vi "SPECAN_AMPM_ACP_TXP.vi"() -> ()   [LabVIEW 2016]
doc: "This example illustrates how to use the RFmx SpecAn and LTE personalities together with the RFSG drivers to perform ACP and EVM measurements with or without digital predistortion (DPD) of the waveform input to the DUT. \n\nDPD is a technique to optimize the operating point of power amplifiers and other non-linear RFIC devices. Power amplifiers are much more efficient if they operate near compression. However, compressing signal amplitudes can significantly deteriorate the amplified signal's quality both, in-band (e.g., EVM increases due to non-linear distortion of the signal's I/Q constellation) and out-of-band (e.g., ACP or SEM test fails due to spectral regrowth). With DPD, the original waveform is first pre-distorted in a way that matches the non-linear effects of the RFIC device before being fed through the device. The resulting output is a much cleaner amplified and/or filtered version of the original waveform. \n\nDifferent DPD models can be used to trade off performance with computational ease, with the Lookup-Table (LUT) model the simplest and the Generalized Memory Polynomial Model (GMP) the most complex. With a LUT, the DPD algorithm achieves gain and phase linearization on average. If you want to correct for memory effects - i.e., an output sample not only depends on the current input but also previous input samples; you will notice that a specific input power value translates into a range of gain and phase values - you would use one of the memory polynomial models. For these models, several parameters such as polynomial order and memory depth are available to fine-tune the model to the DUT behavior."
uses:
  <instrlib>/niRFSG/niRFSG.llb/niRFSG Exported Signal Destinations.ctl
  Source/SG/Typedefs/Instrument Configuration.ctl
  <instrlib>/niRFSG/niRFSG.llb/niRFSG Ref Clock Sources.ctl
  Source/SA/RFmxSpecAn/Typedefs/SpecAn AMPM Configuration.ctl
  Source/SG/Typedefs/Waveform.ctl
  Source/SA/RFmxSpecAn/Typedefs/SpecAn AMPM Results.ctl
  Source/SA/RFmxSpecAn/Typedefs/SpecAn Common Configuration.ctl
  Source/SA/RFmxSpecAn/Typedefs/SpecAn ACP Configuration.ctl
  Source/SA/RFmxSpecAn/Typedefs/SpecAn ACP Carrier Channel Configuration.ctl
  Source/SA/RFmxSpecAn/Typedefs/SpecAn ACP Offset Channel Configuration.ctl
  Source/SA/RFmxSpecAn/Typedefs/SpecAn ACP Offset Results.ctl
  Source/SA/RFmxSpecAn/Typedefs/SpecAn ACP Component Carrier Results.ctl
  Source/SA/RFmxSpecAn/Typedefs/SpecAn TxP Configuration.ctl
  Source/SA/RFmxSpecAn/Typedefs/SpecAn TxP Results.ctl
  <vilib>/RFmx/SpecAn/mx/RFmxSpecAn.llb/RFmxSpecAn Select Measurement (Single).vi
  <vilib>/RFmx/SpecAn/mx/RFmxSpecAn.llb/RFmxSpecAn AMPM Fetch AM to AM Trace.vi
  <vilib>/RFmx/SpecAn/mx/RFmxSpecAn.llb/RFmxSpecAn AMPM Fetch AM to PM Trace.vi
  <vilib>/RFmx/SpecAn/mx/RFmxSpecAn.llb/RFmxSpecAn ACP Fetch Spectrum.vi
  <vilib>/RFmx/SpecAn/mx/RFmxSpecAn.llb/RFmxSpecAn TXP Fetch Power Trace.vi
  Source/SG/SG.lvlib
  Source/SA/RFmxSpecAn/RFmxSpecAn.lvlib
panel:
  in  "Display Tab Control":enum32{"AMPM Results", "ACP Results", "TxP"}(tab)
  out "AM to AM Plot":T1(graph)
  out "AM to PM Plot":T2(graph)
  out "AMPM Measurement Results":T3 {"AM to PM Residual (deg)" format="%.2f"; "AM to AM Residual (dB)" format="%.2f"; "Mean RMS EVM (%)" format="%.2f"; "1 dB Compression Point (dBm)" format="%.2f"; "Mean Linear Gain (dB)" format="%.2f"}
  out "Spectrum":cluster{"x0":dbl, "dx":dbl, "y":sgl[]}(graph) caption="DUT Output Spectrum"
  out "Offset Results":T4[](array[typedef])
  out "Component Carrier Results":T5[](array[typedef])
  out "Total Carrier Power (dBm or dBm/Hz)":dbl
  out "Power Trace":cluster{"x0":dbl, "dx":dbl, "y":sgl[]}(graph)
  out "TxP Results":T6 {"Minimum Power (dBm)" format="%.2f"; "Maximum Power (dBm)" format="%.2f"; "Peak to Average Ratio (dB)" format="%.2f"; "Average Mean Power (dBm)" format="%.2f"}
  in  "Measurement Settings Tab Control":T7(tab)
  in  "TxP Config":T8={"Measurement Interval (s)"=0.001, "RBW (Hz)"=20000000.0, "RBW Filter Type"=5, "RRC Alpha"=0.0, "Averaging Enabled"=0, "Averaging Count"=10, "Averaging Type"=0} {"Averaging Type" items=["RMS", "Log", "Scalar", "Max", "Min"]; "Averaging Enabled" items=["False", "True"]; "RRC Alpha" format="%.3g"; "RBW Filter Type" items=["None"=5, "Gaussian"=1, "Flat"=2, "RRC"=6]; "RBW (Hz)" format="%.3p"; "Measurement Interval (s)" format="%.2p"}
  in  "RFmx SpecAn AMPM Configuration":T9={"Measurement Interval (s)"=0.0001, "DUT Average Input Power (dBm)"=-20.0, "Signal Type"=0, "Reference Waveform"={"Waveform Name"="Wfm", "Waveform"={"x0"=0.0, "dx"=0.0, "y"=[]}, "Signal Bandwidth (Hz)"=0.0, "PAPR (dB)"=0.0, "Burst Length (s)"=0.0, "Sample Rate"=0.0, "Burst Start Locations"=[], "Burst Stop Locations"=[], "Idle Duration Present?"=FALSE, "Runtime Scaling"=0.0}} {"Reference Waveform"."Runtime Scaling" format="%#_6p"; "Reference Waveform"."Sample Rate" format="%#_6p"; "Reference Waveform"."Burst Length (s)" format="%#_6p"; "Reference Waveform"."PAPR (dB)" format="%.2f"; "Reference Waveform"."Signal Bandwidth (Hz)" format="%#_6p"; "Reference Waveform"."Waveform"."y" format="%.2f"; "Reference Waveform"."Waveform"."dx" format="%^.2e"; "Reference Waveform"."Waveform"."x0" format="%^.2e"; "Signal Type" items=["Modulated", "Tones"]; "DUT Average Input Power (dBm)" format="%.2f"; "Measurement Interval (s)" format="%.2p"}
  in  "ACP Configuration":T11={"Power Units"=0, "Averaging Enabled"=0, "Averaging Count"=10, "Averaging Type"=0, "FFT Window"=1, "FFT Padding"=-1.0, "RBW Auto"=1, "RBW (Hz)"=10000.0, "RBW Filter Type"=1, "Sweep Time Auto"=1, "Sweep Time Interval (s)"=0.001, " Carrier Channel Configuration"=[], "Offset Channel Configuration"=[]} {"Offset Channel Configuration"."RRC Alpha" format="%.3g"; "Offset Channel Configuration"."RRC Filter Enabled" items=["False", "True"]; "Offset Channel Configuration"."Relative Attenuation (dB)" format="%.2f"; "Offset Channel Configuration"."Power Reference Carrier" items=["Closest", "Highest", "Composite", "Specific"]; "Offset Channel Configuration"."Sideband" items=["Neg", "Pos", "Both"]; "Offset Channel Configuration"."Frequency (Hz)" format="%.3p"; "Offset Channel Configuration"."Enabled" items=["False", "True"]; "Offset Channel Configuration"."Integration Bandwidth (Hz)" format="%.3p"; "Carrier Channel Configuration"."RRC Alpha" format="%.3g"; "Carrier Channel Configuration"."RRC Filter Enabled" items=["False", "True"]; "Carrier Channel Configuration"."Mode" items=["Passive", "Active"]; "Carrier Channel Configuration"."Frequency (Hz)" format="%.3p"; "Carrier Channel Configuration"."Integration Bandwidth (Hz)" format="%.3p"; "Sweep Time Interval (s)" format="%.2p"; "Sweep Time Auto" items=["False", "True"]; "RBW Filter Type" items=["FFT Based", "Gaussian", "Flat", "Synch Tuned - 4", "Synch Tuned - 5"]; "RBW (Hz)" format="%.3p"; "RBW Auto" items=["False", "True"]; "FFT Padding" format="%.2f"; "FFT Window" items=["None", "Flat Top", "Hanning", "Hamming", "Gaussian", "Blackman", "Blackman-Harris", "Kaiser-Bessel"]; "Averaging Type" items=["RMS", "Log", "Scalar", "Max", "Min", "Vector"]; "Averaging Enabled" items=["False", "True"]; "Power Units" items=["dBm", "dBm/Hz"]}
  in  "Offset Channel Configuration":T13[](array[typedef])=[{"Integration Bandwidth (Hz)"=18000000.0, "Enabled"=1, "Frequency (Hz)"=20000000.0, "Sideband"=2, "Power Reference Carrier"=0, "Power Reference Specific Index"=0, "Relative Attenuation (dB)"=0.0, "RRC Filter Enabled"=0, "RRC Alpha"=0.22}, {"Integration Bandwidth (Hz)"=3840000.0, "Enabled"=1, "Frequency (Hz)"=12500000.0, "Sideband"=2, "Power Reference Carrier"=0, "Power Reference Specific Index"=0, "Relative Attenuation (dB)"=0.0, "RRC Filter Enabled"=0, "RRC Alpha"=0.22}, {"Integration Bandwidth (Hz)"=3840000.0, "Enabled"=1, "Frequency (Hz)"=17500000.0, "Sideband"=2, "Power Reference Carrier"=0, "Power Reference Specific Index"=0, "Relative Attenuation (dB)"=0.0, "RRC Filter Enabled"=0, "RRC Alpha"=0.22}] {"RRC Alpha" format="%.3g"; "RRC Filter Enabled" items=["False", "True"]; "Relative Attenuation (dB)" format="%.2f"; "Power Reference Carrier" items=["Closest", "Highest", "Composite", "Specific"]; "Sideband" items=["Neg", "Pos", "Both"]; "Frequency (Hz)" format="%.3p"; "Enabled" items=["False", "True"]; "Integration Bandwidth (Hz)" format="%.3p"}
  in  "Carrier Channel Configuration":T12[](array[typedef])=[{"Frequency (Hz)"=0.0, "Integration Bandwidth (Hz)"=18000000.0, "Mode"=1, "RRC Filter Enabled"=0, "RRC Alpha"=0.22}] {"RRC Alpha" format="%.3g"; "RRC Filter Enabled" items=["False", "True"]; "Mode" items=["Passive", "Active"]; "Frequency (Hz)" format="%.3p"; "Integration Bandwidth (Hz)" format="%.3p"}
  in  "Resource Control":enum32{"RFSG", "RFSA"}(tab)
  in  "Marker Event Output Terminal":T14="PXI_Trig0"
  in  "Reference Waveform File Path":path=path "C:/Users/Public/Documents/National Instruments/RFIC Test Software/Waveforms/LTE_FDD_UL_1x20MHz_256QAM_OS4.tdms"
  in  "RFSG Resource Name":refnum<k15>="RFSG"
  in  "SG Configuration":T15={"Reference Clock Source"="PXI_CLK", "Carrier Frequency (Hz)"=3500000000.0, "DUT Average Input Power (dBm)"=-10.0, "External Attenuation (dB)"=0.0, "Share LO  SG->SA"=FALSE, "SelectedPorts"=""} {"Carrier Frequency (Hz)" format="%#_6p"}
  in  "RFSA Resource Name":refnum<k15>="RFSA"
  in  "RFmx SpecAn Configuration":T17={"Center Frequency (Hz)"=1000000000.0, "Reference Level (dBm)"=0.0, "External Attenuation (dB)"=0.0, "Enable Trigger?"=TRUE, "Digital Edge Source"="PXI_Trig0", "Digital Edge Type"=0, "Trigger Delay (s)"=0.0, "Frequency Reference Source"="PXI_Clk", "SelectedPorts"="", "Auto Level Enabled"=FALSE, "Auto Level Measurement Interval (s)"=0.01, "Auto Level Bandwidth (Hz)"=20000000.0} {"Auto Level Bandwidth (Hz)" format="%#_6p"; "Auto Level Measurement Interval (s)" format="%#_6p"; "Trigger Delay (s)" format="%.2p"; "Digital Edge Type" items=["Rising Edge", "Falling Edge"]; "External Attenuation (dB)" format="%.2f"; "Reference Level (dBm)" format="%.2f"; "Center Frequency (Hz)" format="%.6p"}
  in  "Center Frequency / SG IF (Hz)":dbl=3500000000.0 format="%.6p"
  in  "Error Tab Control":enum32{"Page 1", "Page 2"}(tab)
  out "error out":errorcluster
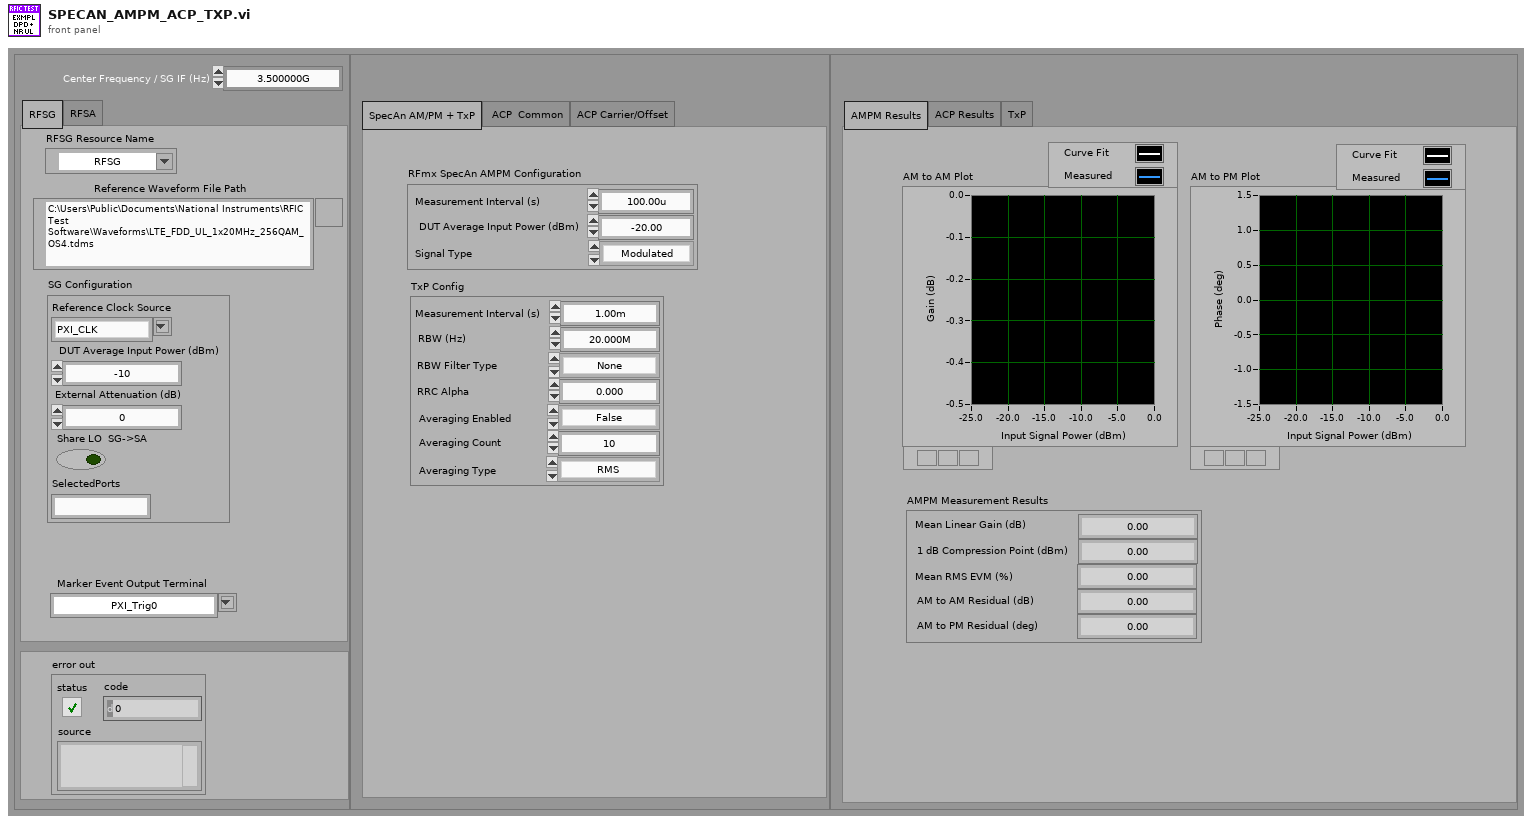
[diagram p1: front panel]
types:
  T1 = cluster{"Input Powers (dBm)":sgl[], "Curve Fit AM to AM (dB)":sgl[]}[]
  T2 = cluster{"Input Powers (dBm)":sgl[], "Curve Fit AM to PM (dB)":sgl[]}[]
  T3 = typedef "RFmxSpecAn.lvlib/SpecAn AMPM Results.ctl" = cluster{"Mean Linear Gain (dB)":dbl, "1 dB Compression Point (dBm)":dbl, "Mean RMS EVM (%)":dbl, "AM to AM Residual (dB)":dbl, "AM to PM Residual (deg)":dbl}
  T4 = typedef "RFmxSpecAn.lvlib/SpecAn ACP Offset Results.ctl" = cluster{"Lower Absolute Power (dBm)":dbl, "Upper Absolute Power (dBm)":dbl, "Lower Relative Power (dB)":dbl, "Upper Relative Power (dB)":dbl, "Offset Frequency (Hz)":dbl, "Offset Integration Bandwidth (Hz)":dbl}
  T5 = typedef "RFmxSpecAn.lvlib/SpecAn ACP Component Carrier Results.ctl" = cluster{"Carrier Frequency (Hz)":dbl, "Integration Bandwidth (Hz)":dbl, "Absolute Power (dBm or dBmHz)":dbl, "Total Relative Power (dB)":dbl}
  T6 = typedef "RFmxSpecAn.lvlib/SpecAn TxP Results.ctl" = cluster{"Average Mean Power (dBm)":dbl, "Peak to Average Ratio (dB)":dbl, "Maximum Power (dBm)":dbl, "Minimum Power (dBm)":dbl}
  T7 = enum32{"SpecAn AM/PM + TxP", " ACP  Common", "ACP Carrier/Offset"}
  T8 = typedef "RFmxSpecAn.lvlib/SpecAn TxP Configuration.ctl" = cluster{"Measurement Interval (s)":dbl, "RBW (Hz)":dbl, "RBW Filter Type":i32, "RRC Alpha":dbl, "Averaging Enabled":i32, "Averaging Count":i32, "Averaging Type":i32}
  T9 = typedef "RFmxSpecAn.lvlib/SpecAn AMPM Configuration.ctl" = cluster{"Measurement Interval (s)":dbl, "DUT Average Input Power (dBm)":dbl, "Signal Type":i32, "Reference Waveform":T10}
  T10 = typedef "SG.lvlib/Waveform.ctl" = cluster{"Waveform Name":string, "Waveform":cluster{"x0":dbl, "dx":dbl, "y":csg[]}, "Signal Bandwidth (Hz)":dbl, "PAPR (dB)":dbl, "Burst Length (s)":dbl, "Sample Rate":dbl, "Burst Start Locations":i32[], "Burst Stop Locations":i32[], "Idle Duration Present?":bool, "Runtime Scaling":dbl}
  T11 = typedef "RFmxSpecAn.lvlib/SpecAn ACP Configuration.ctl" = cluster{"Power Units":i32, "Averaging Enabled":i32, "Averaging Count":i32, "Averaging Type":i32, "FFT Window":i32, "FFT Padding":dbl, "RBW Auto":i32, "RBW (Hz)":dbl, "RBW Filter Type":i32, "Sweep Time Auto":i32, "Sweep Time Interval (s)":dbl, " Carrier Channel Configuration":T12[], "Offset Channel Configuration":T13[]}
  T12 = typedef "RFmxSpecAn.lvlib/SpecAn ACP Carrier Channel Configuration.ctl" = cluster{"Frequency (Hz)":dbl, "Integration Bandwidth (Hz)":dbl, "Mode":i32, "RRC Filter Enabled":i32, "RRC Alpha":dbl}
  T13 = typedef "RFmxSpecAn.lvlib/SpecAn ACP Offset Channel Configuration.ctl" = cluster{"Integration Bandwidth (Hz)":dbl, "Enabled":i32, "Frequency (Hz)":dbl, "Sideband":i32, "Power Reference Carrier":i32, "Power Reference Specific Index":i32, "Relative Attenuation (dB)":dbl, "RRC Filter Enabled":i32, "RRC Alpha":dbl}
  T14 = typedef "niRFSG Exported Signal Destinations.ctl" = string
  T15 = typedef "SG.lvlib/Instrument Configuration.ctl" = cluster{"Reference Clock Source":T16, "Carrier Frequency (Hz)":dbl, "DUT Average Input Power (dBm)":dbl, "External Attenuation (dB)":dbl, "Share LO  SG->SA":bool, "SelectedPorts":string}
  T16 = typedef "niRFSG Ref Clock Sources.ctl" = string
  T17 = typedef "RFmxSpecAn.lvlib/SpecAn Common Configuration.ctl" = cluster{"Center Frequency (Hz)":dbl, "Reference Level (dBm)":dbl, "External Attenuation (dB)":dbl, "Enable Trigger?":bool, "Digital Edge Source":string, "Digital Edge Type":i32, "Trigger Delay (s)":dbl, "Frequency Reference Source":string, "SelectedPorts":string, "Auto Level Enabled":bool, "Auto Level Measurement Interval (s)":dbl, "Auto Level Bandwidth (Hz)":dbl}
  T18 = enum16{"ACP", "CCDF", "CHP", "FCnt", "Harmonics", "OBW", "SEM", "Spectrum", "Spur", "TXP", "AMPM", "DPD", "IQ", "IM", "NF", "PhaseNoise", "PAVT"}
  T19 = enum16{"ACP", "CCDF", "CHP", "FCnt", "Harmonics", "OBW", "SEM", "Spectrum", "Spur", "TXP", "AMPM", "DPD", "IQ", "IM", "NF", "PhaseNoise"}
  T20 = cluster{"Mean Linear Gain (dB)":dbl, "Mean RMS EVM (%)":dbl, "AM to AM Residual (dB)":dbl, "AM to PM Residual (deg)":dbl, "1 dB Compression Point (dBm)":dbl}
  T21 = cluster{"Reference Powers (dBm)":sgl[], "Curve Fit AM to AM (dB)":sgl[]}
  T22 = cluster{"Reference Powers (dBm)":sgl[], "Measured AM to AM (dB)":sgl[]}
  T23 = cluster{"Reference Powers (dBm)":sgl[], "Curve Fit AM to PM (deg)":sgl[]}
  T24 = cluster{"Reference Powers (dBm)":sgl[], "Measured AM to PM (deg)":sgl[]}
  T25 = cluster{"Reference Powers (dBm)":sgl[], "Measured AM to AM (dB)":sgl[]}[]
  T26 = cluster{"Reference Powers (dBm)":sgl[], "Measured AM to PM (deg)":sgl[]}[]
  T27 = typedef "RFmxSpecAn.lvlib/SpecAn ACP Results.ctl" = cluster{"Total Carrier Power (dBm or dBm/Hz)":dbl, "Offset Results":T4[], "Component Carrier Results":T5[]}
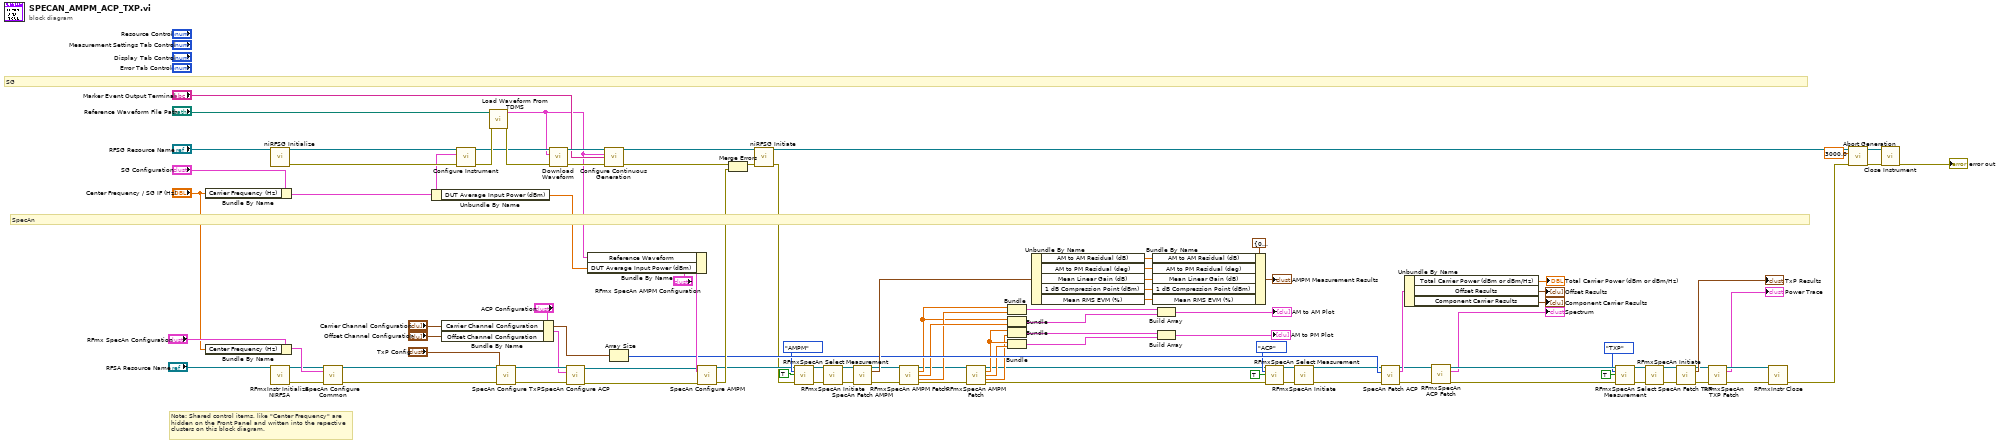
[diagram p0: block diagram]
diagram:
  # "Note: Shared control items, like \"Center Frequency\" are \nhidden on the Front Panel and written into the repective \nclusters on this block diagram."
  # "SG"
  # "SpecAn"
  n1 = Bundle By Name(cluster="SG Configuration", "Carrier Frequency (Hz)"="Center Frequency / SG IF (Hz)") -> (w82:T15)
  n2 = Bundle By Name(cluster="RFmx SpecAn Configuration", "Center Frequency (Hz)"="Center Frequency / SG IF (Hz)") -> (w63:T17)
  n3 = call <instrlib>:"niRFSG Initialize.vi"("resource name"="RFSG Resource Name") -> ("instrument handle"=w98:refnum<k15>, "error out"=w97:errorcluster)  [unwired: 13 in]
  n4 = call <vilib>:"RFmxInstr Initialize NIRFSA.vi"("Resource Name"="RFSA Resource Name") -> ("Instrument Handle Out"=w32:refnum<k21>, "error out"=w31:errorcluster)  [unwired: 12 in, 1 out]
  n5 = call "SpecAn Configure Common.vi"("RFmx Handle In"=w32, "SpecAn Common Configuration"=w63, "error in (no error)"=w31) -> ("RFmx Handle Out"=w61:refnum<k21>, "error out"=w59:errorcluster)  [unwired: 11 in]
  n6 = Unbundle By Name(w82) -> ("DUT Average Input Power (dBm)"=w81:dbl)
  n7 = Bundle By Name(cluster="ACP Configuration", "Carrier Channel Configuration"="Carrier Channel Configuration", "Offset Channel Configuration"="Offset Channel Configuration") -> (w34:T11)
  n8 = call "Configure Instrument.vi"("RFSG Session In"=w98, "SG Configuration"=w82, "error in (no error)"=w97) -> ("RFSG Session Out"=w103:refnum<k15>, "error out"=w105:errorcluster)  [unwired: 11 in]
  n9 = call "Load Waveform From TDMS.vi"("TDMS File Path"="Reference Waveform File Path", "error in (no error)"=w105) -> ("Waveform"=w35:T10, "error out"=w104:errorcluster)  [unwired: 12 in]
  n10 = call "SpecAn Configure TxP.vi"("Instrument Handle In"=w61, "TxP Config"="TxP Config", "error in (no error)"=w59) -> ("Instrument Handle Out"=w60:refnum<k21>, "error out"=w58:errorcluster)  [unwired: 11 in]
  n11 = call "Download Waveform.vi"("RFSG handle"=w103, "Waveform In"=w35, "error in (no error)"=w104) -> ("RFSG handle out"=w96:refnum<k15>, "error out"=w94:errorcluster)  [unwired: 11 in]
  n12 = call "SpecAn Configure ACP.vi"("Instrument Handle In"=w60, "ACP Configuration"=w34, "error in (no error)"=w58) -> ("Instrument Handle Out"=w68:refnum<k21>, "error out"=w67:errorcluster)  [unwired: 11 in]
  n13 = Bundle By Name(cluster="RFmx SpecAn AMPM Configuration", "Reference Waveform"=w35, "DUT Average Input Power (dBm)"=w81) -> (w83:T9)
  n14 = call "Configure Continuous Generation.vi"("RFSG handle"=w96, "Waveform"=w35, "Waveform Start Trigger Export"="Marker Event Output Terminal", "error in"=w94) -> ("RFSG handle out"=w95:refnum<k15>, "error out"=w93:errorcluster)  [unwired: 10 in]
  n15 = Array Size(array="Carrier Channel Configuration") -> (size(s)=w64:i32)
  n16 = call "SpecAn Configure AMPM.vi"("RFmx Handle In"=w68, "RFmx SpecAn AMPM Configuration"=w83, "error in (no error)"=w67) -> ("RFmx Handle Out"=w45:refnum<k21>, "error out"=w85:errorcluster)  [unwired: 11 in]
  n17 = Merge Errors(w93, w85) -> (w92:errorcluster)
  n18 = call <instrlib>:"niRFSG Initiate.vi"("instrument handle"=w95, "error in"=w92) -> ("instrument handle out"=w102:refnum<k15>, "error out"=w44:errorcluster)  [unwired: 12 in]
  n19 = call-poly <vilib>:"RFmxSpecAn Select Measurement.vi"("Instrument Handle In"=w45, "Measurement"=T19."AMPM", "Enable All Traces"=TRUE, "error in (no error)"=w44) -> ("Instrument Handle Out"=w53:refnum<k21>, "error out"=w54:errorcluster)  [unwired: 10 in]
  n20 = call <vilib>:"RFmxSpecAn Initiate.vi"("Instrument Handle In"=w53, "error in (no error)"=w54) -> ("Instrument Handle Out"=w41:refnum<k21>, "error out"=w43:errorcluster)  [unwired: 11 in, 1 out]
  n21 = call "SpecAn Fetch AMPM.vi"("RFmx Handle In"=w41, "error in (no error)"=w43) -> ("RFmx Handle Out"=w22:refnum<k21>, "AMPM Results"=w79:T3, "error out"=w19:errorcluster)  [unwired: 11 in]
  n22 = call-poly <vilib>:"RFmxSpecAn AMPM Fetch.vi"("Instrument Handle In"=w22, "error in (no error)"=w19) -> ("Instrument Handle Out"=w20:refnum<k21>, "Reference Powers (dBm)"=w26:sgl[], "Measured AM to AM (dB)"=w28:sgl[], "Curve Fit AM to AM (dB)"=w27:sgl[], "error out"=w17:errorcluster)  [unwired: 9 in]
  n23 = call-poly <vilib>:"RFmxSpecAn AMPM Fetch.vi"("Instrument Handle In"=w20, "error in (no error)"=w17) -> ("Instrument Handle Out"=w21:refnum<k21>, "Reference Powers (dBm)"=w25:sgl[], "Measured AM to PM (deg)"=w24:sgl[], "Curve Fit AM to PM (deg)"=w23:sgl[], "error out"=w18:errorcluster)  [unwired: 9 in]
  n24 = Bundle("Reference Powers (dBm)"=w26, "Curve Fit AM to AM (dB)"=w27) -> (w16:T21)  [unwired: 1 in]
  n25 = Bundle("Reference Powers (dBm)"=w26, "Measured AM to AM (dB)"=w28) -> (w15:T22)  [unwired: 1 in]
  n26 = Bundle("Reference Powers (dBm)"=w25, "Curve Fit AM to PM (deg)"=w23) -> (w13:T23)  [unwired: 1 in]
  n27 = Bundle("Reference Powers (dBm)"=w25, "Measured AM to PM (deg)"=w24) -> (w14:T24)  [unwired: 1 in]
  n28 = Unbundle By Name(w79) -> ("AM to AM Residual (dB)"=w78:dbl, "AM to PM Residual (deg)"=w77:dbl, "Mean Linear Gain (dB)"=w75:dbl, "1 dB Compression Point (dBm)"=w74:dbl, "Mean RMS EVM (%)"=w73:dbl)
  n29 = Bundle By Name(cluster=T20 {"Mean Linear Gain (dB)"=0.0, "Mean RMS EVM (%)"=0.0, "AM to AM Residual (dB)"=0.0, "AM to PM Residual (deg)"=0.0, "1 dB Compression Point (dBm)"=0.0} ("Measurement"), "AM to AM Residual (dB)"=w78, "AM to PM Residual (deg)"=w77, "Mean Linear Gain (dB)"=w75, "1 dB Compression Point (dBm)"=w74, "Mean RMS EVM (%)"=w73) -> (→"AMPM Measurement Results":T20)
  n30 = Build Array(w16, w15) -> (→"AM to AM Plot":T25)
  n31 = Build Array(w13, w14) -> (→"AM to PM Plot":T26)
  n32 = call-poly <vilib>:"RFmxSpecAn Select Measurement.vi"("Instrument Handle In"=w21, "Measurement"=T19."ACP", "Enable All Traces"=TRUE, "error in (no error)"=w18) -> ("Instrument Handle Out"=w49:refnum<k21>, "error out"=w50:errorcluster)  [unwired: 10 in]
  n33 = call <vilib>:"RFmxSpecAn Initiate.vi"("Instrument Handle In"=w49, "error in (no error)"=w50) -> ("Instrument Handle Out"=w40:refnum<k21>, "error out"=w42:errorcluster)  [unwired: 11 in, 1 out]
  n34 = call "SpecAn Fetch ACP.vi"("RFmx Handle In"=w40, "Num Carrier Channels"=w64, "error in (no error)"=w42) -> ("RFmx Handle Out"=w12:refnum<k21>, "ACP Results"=w66:T27, "error out"=w11:errorcluster)  [unwired: 10 in]
  n35 = Unbundle By Name(w66) -> ("Total Carrier Power (dBm or dBm/Hz)"=→"Total Carrier Power (dBm or dBm/Hz)":dbl, "Offset Results"=→"Offset Results":T4[], "Component Carrier Results"=→"Component Carrier Results":T5[])
  n36 = call-poly <vilib>:"RFmxSpecAn ACP Fetch.vi"("Instrument Handle In"=w12, "error in (no error)"=w11) -> ("Instrument Handle Out"=w9:refnum<k21>, "Spectrum (dBm or dBm/Hz)"=→"Spectrum":cluster{"x0":dbl, "dx":dbl, "y":sgl[]}, "error out"=w10:errorcluster)  [unwired: 11 in]
  n37 = call-poly <vilib>:"RFmxSpecAn Select Measurement.vi"("Instrument Handle In"=w9, "Measurement"=T18."TXP", "Enable All Traces"=TRUE, "error in (no error)"=w10) -> ("Instrument Handle Out"=w46:refnum<k21>, "error out"=w47:errorcluster)  [unwired: 10 in]
  n38 = call <vilib>:"RFmxSpecAn Initiate.vi"("Instrument Handle In"=w46, "error in (no error)"=w47) -> ("Instrument Handle Out"=w39:refnum<k21>, "error out"=w37:errorcluster)  [unwired: 11 in, 1 out]
  n39 = call "SpecAn Fetch TxP.vi"("Instrument Handle In"=w39, "error in (no error)"=w37) -> ("Instrument Handle Out"=w7:refnum<k21>, "TxP Results"=→"TxP Results":T6, "error out"=w5:errorcluster)  [unwired: 11 in]
  n40 = call-poly <vilib>:"RFmxSpecAn TXP Fetch.vi"("Instrument Handle In"=w7, "error in (no error)"=w5) -> ("Instrument Handle Out"=w6:refnum<k21>, "Power (dBm)"=→"Power Trace":cluster{"x0":dbl, "dx":dbl, "y":sgl[]}, "error out"=w4:errorcluster)  [unwired: 11 in]
  n41 = call <vilib>:"RFmxInstr Close.vi"("Instrument Handle In"=w6, "error in (no error)"=w4) -> ("error out"=w86:errorcluster)  [unwired: 13 in]
  n42 = call "Abort Generation.vi"("RFSG handle"=w102, "Timeout (ms)"=3000.0, "error in (no error)"=w86) -> ("RFSG handle out"=w101:refnum<k15>, "error out"=w100:errorcluster)  [unwired: 11 in]
  n43 = call "Close Instrument.vi"("RFSG Handle"=w101, "error in (no error)"=w100) -> ("error out"=→"error out":errorcluster)  [unwired: 13 in]
